vi "Simple Add.vi"() -> ()   [LabVIEW 2015]
panel:
  in  "Numerisch 4":dbl
  out "Numerisch 3":dbl
  in  "Numerisch 2":dbl
  in  "Numerisch":dbl
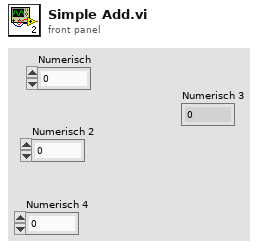
[diagram p1: front panel]
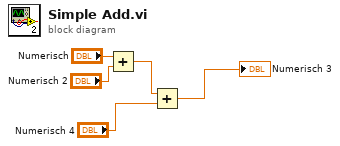
[diagram p0: block diagram]
diagram:
  n1 = Add(x="Numerisch", y="Numerisch 2") -> (x+y=w2:dbl)
  n2 = Add(x=w2, y="Numerisch 4") -> (x+y=→"Numerisch 3":dbl)
